vi "midi_in.recieve_message.vi"(8 "error in (no error)":errorcluster, 11 "LabVIEW-MIDI-XPLAT in":refnum<class "LabVIEW-MIDI-XPLAT.lvclass">) -> (0 "error out":errorcluster, 1 "Return":i32, 2 "buffer":u8[](array[numeric]), 3 "LabVIEW-MIDI-XPLAT out":refnum<class "LabVIEW-MIDI-XPLAT.lvclass">)   [LabVIEW 2020, in "LabVIEW-MIDI-XPLAT.lvclass"]
uses:
  LabVIEW-MIDI-XPLAT.lvclass
  LabVIEW-MIDI-XPLAT.lvclass/LabVIEW-MIDI-XPLAT.ctl
panel:
  out "message_length":i32
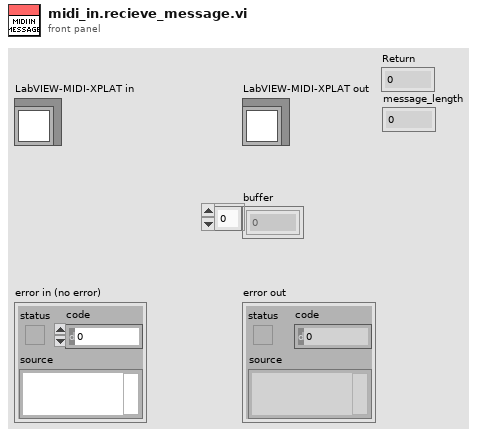
[diagram p1: front panel]
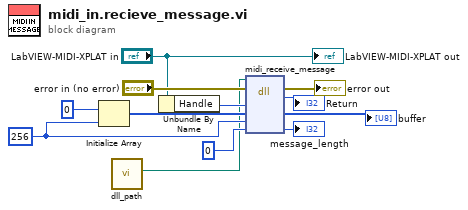
[diagram p0: block diagram]
diagram:
  w6 = 256 ("buffer_size")
  n1 = Initialize Array(u8 0, w6) -> (w5:u8[])
  n2 = call "dll_path.vi"() -> ("dll"=w1:path)  [unwired: 11 in]
  n3 = Unbundle By Name("LabVIEW-MIDI-XPLAT in") -> ("Handle"=w9:i32)
  n4 = dll-call lib="C:/code/LabVIEW-MIDI-XPLAT/dist/TomMIDIllan_*.*" fn="midi_receive_message"(path in=w1, error in="error in (no error)", "handle"=w9, "buffer"=w5, "buffer_size"=w6, "message_length"=0) -> (error out=→"error out":errorcluster, "Return"=→"Return":i32, "buffer"=→"buffer":u8[], "message_length"=→"message_length":i32)  [unwired: 3 in, 1 out]
  "LabVIEW-MIDI-XPLAT out" <- "LabVIEW-MIDI-XPLAT in"
